vi "Time Scale Calibration.vi"(4 "Numeric":i32) -> (0 "max time":dbl, 1 "Time Scale Multiplier":dbl)   [LabVIEW 2012]
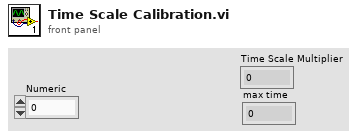
[diagram p1: front panel]
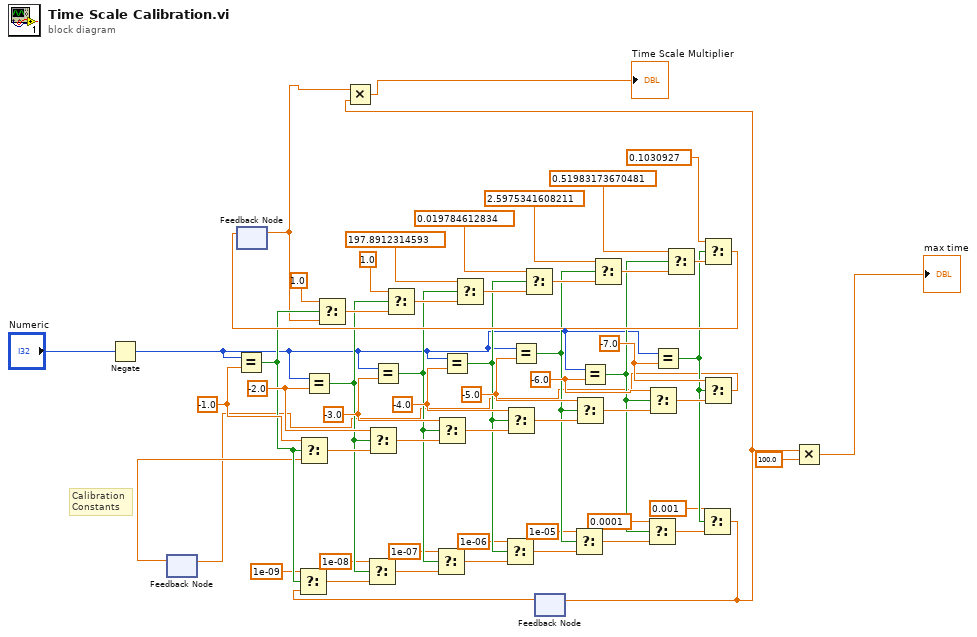
[diagram p0: block diagram]
diagram:
  w50 = -1.0 ("y")
  w51 = -2.0 ("y")
  w52 = -3.0 ("y")
  w53 = -4.0 ("y")
  w54 = -5.0 ("y")
  w55 = -6.0 ("y")
  w56 = -7.0 ("y")
  # "Calibration\nConstants"
  n1 = Negate(x="Numeric") -> (-x=w7:i32)
  n2 = feedback #1() -> (w6:dbl)  [unwired: 1 in]
  n3 = Equal?(x=w7, y=w50) -> (x = y?=w24:bool)
  n4 = feedback #2() -> (w5:dbl)  [unwired: 1 in]
  n5 = Select(t=w50, s=w24, f=w6) -> (s? t:f=w32:dbl)
  n6 = Equal?(x=w7, y=w51) -> (x = y?=w25:bool)
  n7 = Select(t=1.0, s=w24, f=w5) -> (s? t:f=w38:dbl)
  n8 = Select(t=w51, s=w25, f=w32) -> (s? t:f=w33:dbl)
  n9 = Equal?(x=w7, y=w52) -> (x = y?=w26:bool)
  n10 = Select(t=1.0, s=w25, f=w38) -> (s? t:f=w39:dbl)
  n11 = Select(t=w52, s=w26, f=w33) -> (s? t:f=w34:dbl)
  n12 = Equal?(x=w7, y=w53) -> (x = y?=w27:bool)
  n13 = Select(t=197.8912314593, s=w26, f=w39) -> (s? t:f=w40:dbl)
  n14 = Select(t=w53, s=w27, f=w34) -> (s? t:f=w35:dbl)
  n15 = Equal?(x=w7, y=w54) -> (x = y?=w28:bool)
  n16 = Select(t=0.019784612834, s=w27, f=w40) -> (s? t:f=w41:dbl)
  n17 = feedback #3() -> (w10:dbl)  [unwired: 1 in]
  n18 = Select(t=1e-09, s=w24, f=w10) -> (s? t:f=w11:dbl)
  n19 = Select(t=1e-08, s=w25, f=w11) -> (s? t:f=w12:dbl)
  n20 = Select(t=1e-07, s=w26, f=w12) -> (s? t:f=w13:dbl)
  n21 = Select(t=1e-06, s=w27, f=w13) -> (s? t:f=w14:dbl)
  n22 = Select(t=1e-05, s=w28, f=w14) -> (s? t:f=w15:dbl)
  n23 = Select(t=w54, s=w28, f=w35) -> (s? t:f=w36:dbl)
  n24 = Equal?(x=w7, y=w55) -> (x = y?=w29:bool)
  n25 = Select(t=2.5975341608211, s=w28, f=w41) -> (s? t:f=w42:dbl)
  n26 = Select(t=0.0001, s=w29, f=w15) -> (s? t:f=w16:dbl)
  n27 = Select(t=w55, s=w29, f=w36) -> (s? t:f=w37:dbl)
  n28 = Equal?(x=w7, y=w56) -> (x = y?=w30:bool)
  n29 = Select(t=0.51983173670481, s=w29, f=w42) -> (s? t:f=w43:dbl)
  n30 = Select(t=0.001, s=w30, f=w16) -> (s? t:f=w3:dbl)
  n31 = Multiply(x=w5, y=w3) -> (x*y=→"Time Scale Multiplier":dbl)
  n32 = feedback-in #3(w3) -> ()
  n33 = Select(t=0.1030927, s=w30, f=w43) -> (s? t:f=w31:dbl)
  n34 = feedback-in #2(w31) -> ()
  n35 = Select(t=w56, s=w30, f=w37) -> (s? t:f=w4:dbl)
  n36 = feedback-in #1(w4) -> ()
  n37 = Multiply(x=w3, y=100.0) -> (x*y=→"max time":dbl)
